vi "Autonomous Independent.vi"() -> ()   [LabVIEW 2015]
doc: "This VI is called when autonomous begins, and will automatically be terminated when autonomous ends. You can carry out timed or sensor driven robot movement independently without needing to return to the caller."
uses:
  <vilib>/Rock Robotics/WPI/Solenoid/WPI_SolenoidValue.ctl
  <vilib>/Rock Robotics/WPI/CAN/TalonSRX/WPI_CANTalonSRX_APIControlMode.ctl
  <vilib>/Rock Robotics/WPI/Utilities/WPI_GetSetVariantRefNum.vi
  <vilib>/Rock Robotics/Network Tables/NT Write Numeric Array.vi
  <vilib>/Rock Robotics/Network Tables/NT Read String.vi
  <vilib>/Rock Robotics/WPI/RobotDrive/WPI_RobotDriveArcadeDrive_Standard(NoSaturation).vi
  <vilib>/Rock Robotics/Network Tables/NT Write Boolean.vi
  <vilib>/Rock Robotics/WPI/Solenoid/WPI_SolenoidSetEnum.vi
  <vilib>/Rock Robotics/Network Tables/NT Read Number.vi
  Distance.vi
panel:
  out "Current Movement, for debugging":T1 {"Y Joystick Value" scale=1.0..-1.0; "X Joystick Value" scale=-1.0..1.0}
  in  "Array of robot movements":T2(array[cluster])=[{"X Joystick Value"=0.39393939393939403, "Y Joystick Value"=0.0, "Delay (sec)"=1.0, "Movement Name"="turn"}, {"X Joystick Value"=-0.3737373737373737, "Y Joystick Value"=0.0, "Delay (sec)"=1.0, "Movement Name"="turn back"}] {"Y Joystick Value" scale=1.0..-1.0; "X Joystick Value" scale=-1.0..1.0}
  # "Be sure to right-click and choose Data Operations>>Make Current Value default if you want to save the array values with the VI"
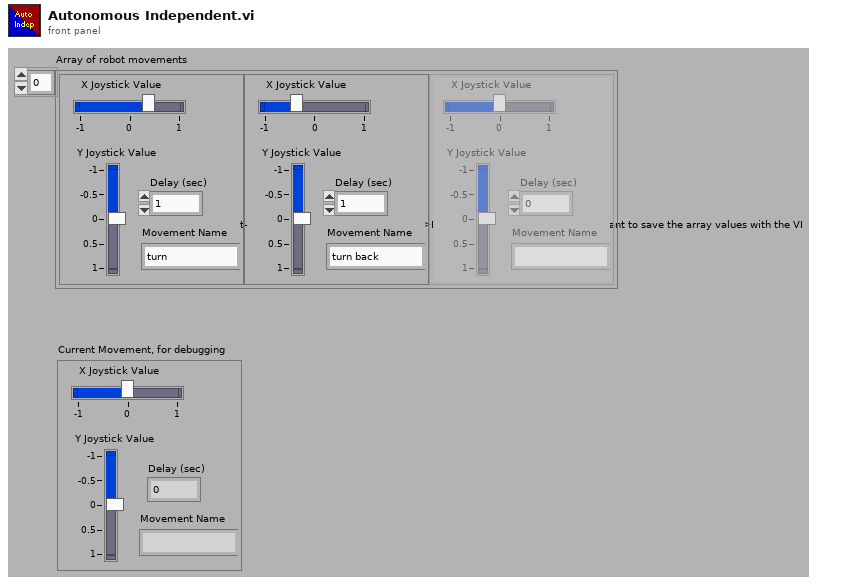
[diagram p1: front panel]
types:
  T1 = cluster{"X Joystick Value":dbl, "Y Joystick Value":dbl, "Delay (sec)":dbl, "Movement Name":string}
  T2 = cluster{"X Joystick Value":dbl, "Y Joystick Value":dbl, "Delay (sec)":dbl, "Movement Name":string}[]
  T3 = typedef "WPI_JoystickDevRef.ctl" = cluster{"Device":T4}
  T4 = typedef "WPI_JoystickDeviceEnum.ctl" = enum16{"USB 0", "USB 1", "USB 2", "USB 3", "USB 4", "USB 5"}
  T5 = typedef "WPI_SolenoidValue.ctl" = enum16{"Off", "On", "Forward", "Reverse"}
  T6 = typedef "WPI_RobotDriveDevRef.ctl" = cluster{"DevStatus":errorcluster, "Motors[]":T7[], "Square Inputs":bool, "Max Output":dbl}
  T7 = typedef "WPI_MotorControlDeviceRef.ctl" = cluster{"DeviceStatus":errorcluster, "Type":T8, "PWM":cluster{"PWM Channel":T9, "DeadBand":T10}, "CAN":cluster{"Device Number":u8, "Control Mode":T11, "Semaphore":T12, "Max Vout":dbl, "TalonSRX Control Mode":T13}, "Invert":bool}
  T8 = typedef "WPI_MotorControlType.ctl" = enum16{"PWM", "CAN", "CANTalonSRX"}
  T9 = typedef "FPGA_DIOPWMChannel.ctl" = enum8{"PWM 0", "PWM 1", "PWM 2", "PWM 3", "PWM 4", "PWM 5", "PWM 6", "PWM 7", "PWM 8", "PWM 9", "PWM MXP 0", "PWM MXP 1", "PWM MXP 2", "PWM MXP 3", "PWM MXP 4", "PWM MXP 5", "PWM MXP 6", "PWM MXP 7", "PWM MXP 8", "PWM MXP 9", "Invalid"}
  T10 = typedef "WPI_PWMDeadband.ctl" = cluster{"Name":string, "maxPositivePwm":i32, "minPositivePwm":i32, "centerPwm":i32, "maxNegativePwm":i32, "minNegativePwm":i32, "angularRange":u16}
  T11 = typedef "WPI_CANJaguar_ControlMode.ctl" = enum8{"Percent VBus", "Current", "Speed", "Position", "Voltage"}
  T12 = typedef "Semaphore RefNum" = refnum<k1>
  T13 = typedef "WPI_CANTalonSRX_APIControlMode.ctl" = enum8{"Percent VBus", "Speed", "Position", "Slave", "Unchanged / Invalid", "Voltage Compensation", "Current", "Motion Profile"}
  T14 = typedef "WPI_SolenoidDevRef.ctl" = cluster{"DevStatus":errorcluster, "Pneumatics Control Module":u8, "Forward Solenoid Channel":T15, "Reverse Solenoid Channel":T15}
  T15 = typedef "WPI_SolenoidChannel.ctl" = enum8{"Solenoid 0", "Solenoid 1", "Solenoid 2", "Solenoid 3", "Solenoid 4", "Solenoid 5", "Solenoid 6", "Solenoid 7", "Invalid"}
  T16 = typedef "WPI_ServoDeviceRef.ctl" = cluster{"DeviceStatus":errorcluster, "PWM Channel":T9, "DeadBand":T10}
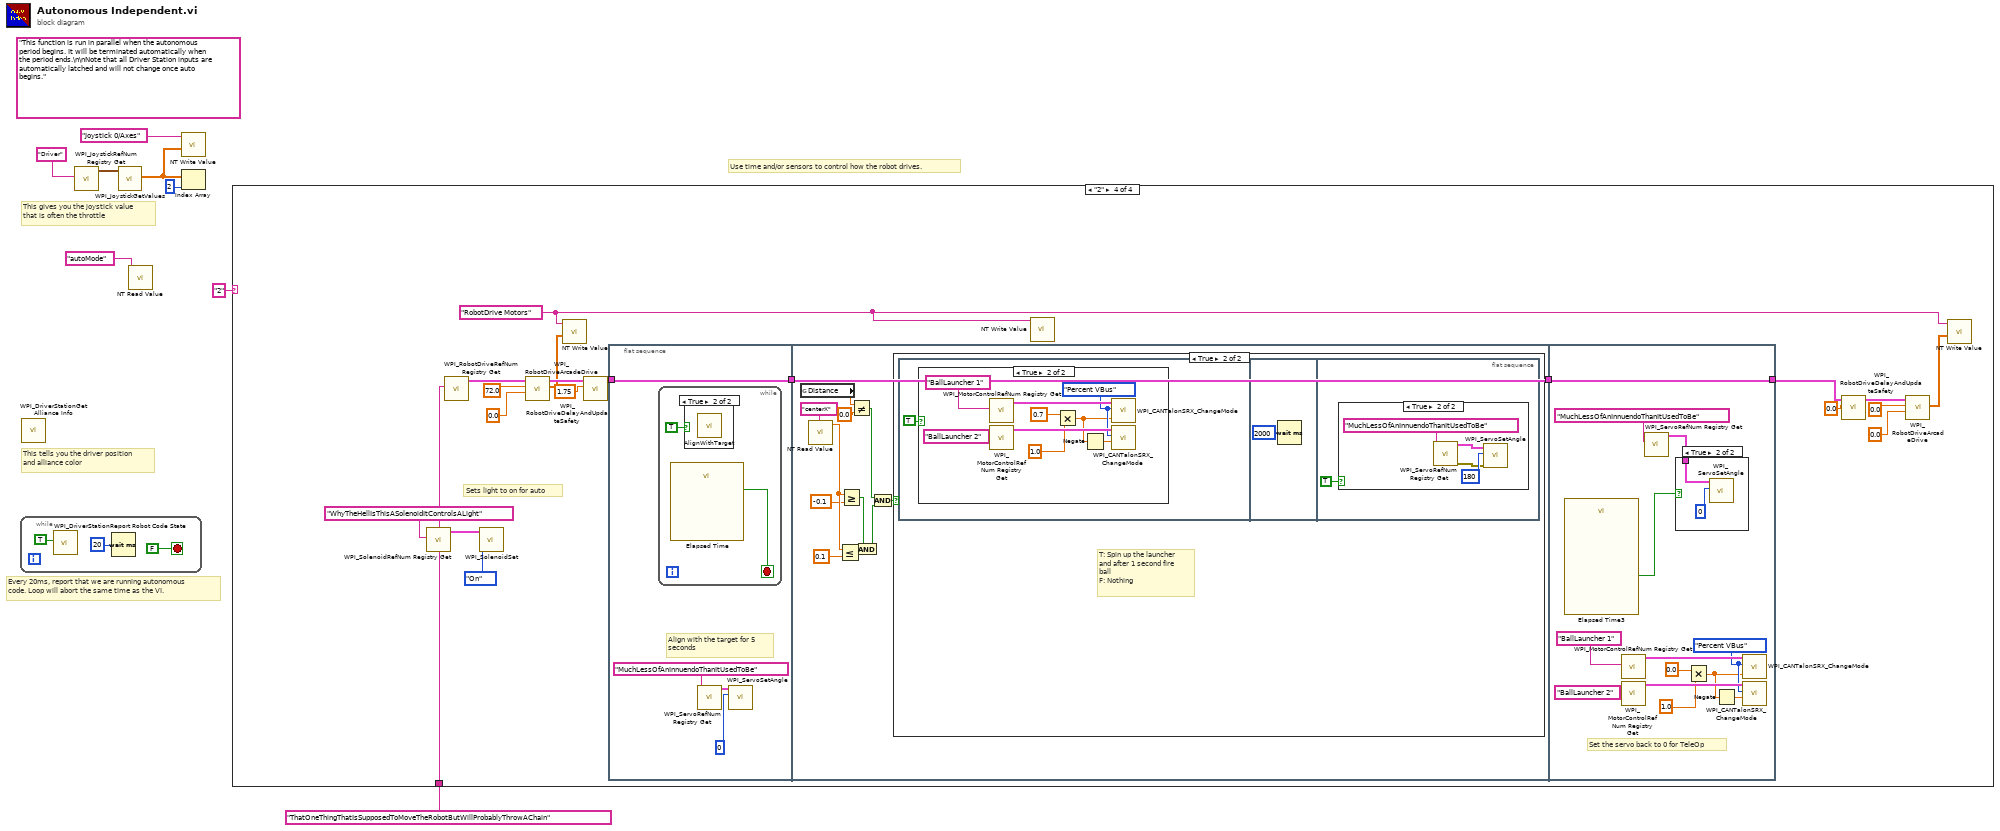
[diagram p0: block diagram]
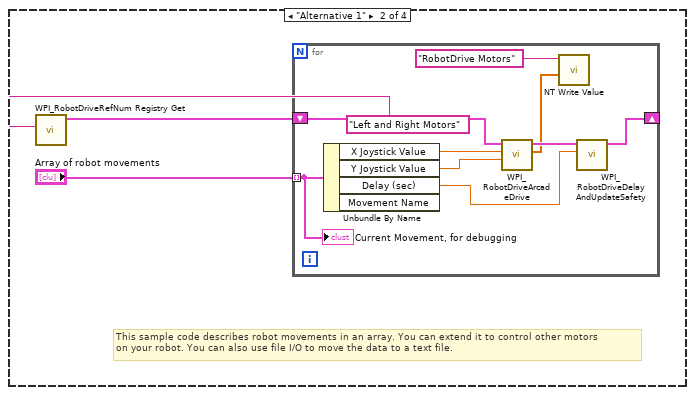
[diagram p3: hidden frame]
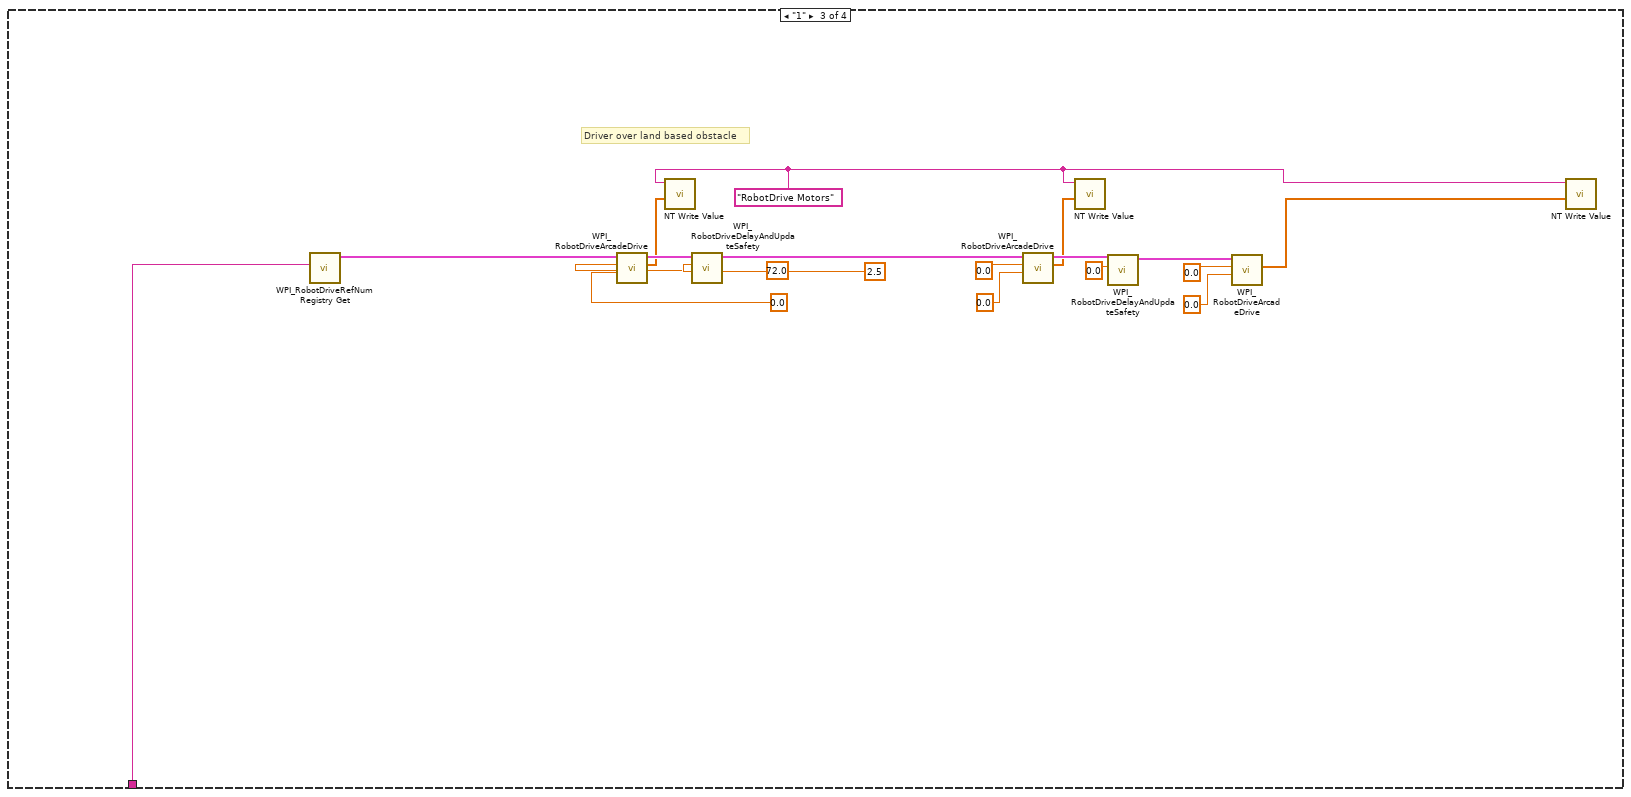
[diagram p4: hidden frame]
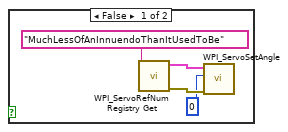
[diagram p8: hidden frame]
diagram:
  (unwired) "This function is run in parallel when the autonomous period begins. It will be terminated automatically when the period ends.\n\nNote that all Driver Station inputs are automatically latched and will not change once auto begins."
  # "Every 20ms, report that we are running autonomous\ncode. Loop will abort the same time as the VI."
  # "This gives you the joystick value\nthat is often the throttle"
  # "Use time and/or sensors to control how the robot drives."
  # "This tells you the driver position\nand alliance color"
  n1 = while {
    stop <- FALSE stop-if-true
    n2 = call <vilib>:"WPI_DriverStationReport Robot Code State.vi"("Autonomous"=TRUE) -> ()  [unwired: 10 in, 1 out]
    n3 = Wait (ms)(milliseconds to wait=u32 20) -> ()  [unwired: 1 out]
  }
  n4 = call <vilib>:"WPI_DriverStationGet Alliance Info.vi"() -> ()  [unwired: 12 out]
  n5 = call <vilib>:"WPI_JoystickRefNum Registry Get.vi"("refnum name"="Driver") -> ("JoystickDevRef"=w7:T3)  [unwired: 1 in, 9 out]
  n6 = call <vilib>:"WPI_JoystickGetValues.vi"("JoystickDevRef"=w7) -> ("Axes"=w5:dbl[])  [unwired: 6 in, 4 out]
  n7 = call-poly <vilib>:"NT Read Value.vi"("Name"="autoMode") -> ()  [unwired: 9 in, 2 out]
  n8 = call-poly <vilib>:"NT Write Value.vi"("Numeric Array"=w5, "Name"="Joystick 0/Axes") -> ()  [unwired: 9 in, 1 out]
  n9 = Index Array(array=w5, index=2) -> ()  [unwired: 1 out]
  n10 = case shown="\"2\"" "2" {
    tunnel: "ThatOneThingThatIsSupposedToMoveTheRobotButWillProbablyThrowAChain" ("refnum name") -> [_ _ w24 w49]
    frame Default {
      # "You can put your main auto here, or you can right-click on the case and make any\nother frame be the default case."
      # "This is the frame that will execute if no selection is made, or if it is not recognized"
    }
    frame "Alternative 1" {
      # "This sample code describes robot movements in an array. You can extend it to control other motors\non your robot. You can also use file I/O to move the data to a text file."
      n11 = call <vilib>:"WPI_RobotDriveRefNum Registry Get.vi"("refnum name"="Left and Right Motors") -> ("RobotDriveDevRef"=w13:T6)  [unwired: 1 in, 9 out]
      n12 = for {
        shift-right: [w21] -> _
        shift-left: w13 -> [w22]
        tunnel: "Array of robot movements" -> [w17] mode=indexing
        n13 = Unbundle By Name(w17) -> ("X Joystick Value"=w20:dbl, "Y Joystick Value"=w19:dbl, "Delay (sec)"=w18:dbl)  [unwired: 1 out]
        n14 = call-poly <vilib>:"WPI_RobotDriveArcadeDrive.vi"("Y axis value"=w19, "X axis value"=w20, "RobotDriveDevRef"=w22) -> ("Motor Values"=w15:dbl[], "RobotDriveDevRef"=w23:T6)  [unwired: 1 in, 6 out]
        n15 = call-poly <vilib>:"NT Write Value.vi"("Numeric Array"=w15, "Name"="RobotDrive Motors") -> ()  [unwired: 9 in, 1 out]
        n16 = call <vilib>:"WPI_RobotDriveDelayAndUpdateSafety.vi"("Delay (s)"=w18, "RobotDriveDevRef"=w23) -> ("RobotDriveDevRef 2"=w21:T6)  [unwired: 8 in, 1 out]
        "Current Movement, for debugging" <- w17
      }
    }
    frame "1" {
      w26 = "RobotDrive Motors" ("Name")
      # "Driver over land based obstacle"
      n17 = call <vilib>:"WPI_RobotDriveRefNum Registry Get.vi"("refnum name"=w24) -> ("RobotDriveDevRef"=w41:T6)  [unwired: 1 in, 9 out]
      n18 = call-poly <vilib>:"WPI_RobotDriveArcadeDrive.vi"("Y axis value"=0.0 ("X axis value"), "X axis value"=72.0, "RobotDriveDevRef"=w41) -> ("Motor Values"=w25:dbl[], "RobotDriveDevRef"=w35:T6)  [unwired: 1 in, 6 out]
      n19 = call-poly <vilib>:"NT Write Value.vi"("Numeric Array"=w25, "Name"=w26) -> ()  [unwired: 9 in, 1 out]
      n20 = call <vilib>:"WPI_RobotDriveDelayAndUpdateSafety.vi"("Delay (s)"=2.5, "RobotDriveDevRef"=w35) -> ("RobotDriveDevRef 2"=w36:T6)  [unwired: 8 in, 1 out]
      n21 = call-poly <vilib>:"WPI_RobotDriveArcadeDrive.vi"("Y axis value"=0.0 ("X axis value"), "X axis value"=0.0, "RobotDriveDevRef"=w36) -> ("Motor Values"=w27:dbl[], "RobotDriveDevRef"=w37:T6)  [unwired: 1 in, 6 out]
      n22 = call-poly <vilib>:"NT Write Value.vi"("Numeric Array"=w27, "Name"=w26) -> ()  [unwired: 9 in, 1 out]
      n23 = call <vilib>:"WPI_RobotDriveDelayAndUpdateSafety.vi"("Delay (s)"=0.0, "RobotDriveDevRef"=w37) -> ("RobotDriveDevRef 2"=w38:T6)  [unwired: 8 in, 1 out]
      n24 = call-poly <vilib>:"WPI_RobotDriveArcadeDrive.vi"("Y axis value"=0.0 ("X axis value"), "X axis value"=0.0, "RobotDriveDevRef"=w38) -> ("Motor Values"=w28:dbl[])  [unwired: 1 in, 7 out]
      n25 = call-poly <vilib>:"NT Write Value.vi"("Numeric Array"=w28, "Name"=w26) -> ()  [unwired: 9 in, 1 out]
    }
    frame "2" {
      w51 = "RobotDrive Motors" ("Name")
      # "Sets light to on for auto"
      n26 = call <vilib>:"WPI_SolenoidRefNum Registry Get.vi"("refnum name"="WhyTheHellIsThisASolenoidItControlsALight") -> ("SolenoidDevRef"=w43:T14)  [unwired: 9 in, 1 out]
      n27 = call <vilib>:"WPI_RobotDriveRefNum Registry Get.vi"("refnum name"=w49) -> ("RobotDriveDevRef"=w61:T6)  [unwired: 1 in, 9 out]
      n28 = call-poly <vilib>:"WPI_SolenoidSet.vi"("Value"=WPI_SolenoidValue."On", "SolenoidDevRef"=w43) -> ()  [unwired: 8 in, 2 out]
      n29 = call-poly <vilib>:"WPI_RobotDriveArcadeDrive.vi"("Y axis value"=0.0 ("X axis value"), "X axis value"=72.0, "RobotDriveDevRef"=w61) -> ("Motor Values"=w50:dbl[], "RobotDriveDevRef"=w57:T6)  [unwired: 1 in, 6 out]
      n30 = call-poly <vilib>:"NT Write Value.vi"("Numeric Array"=w50, "Name"=w51) -> ()  [unwired: 9 in, 1 out]
      n31 = call <vilib>:"WPI_RobotDriveDelayAndUpdateSafety.vi"("Delay (s)"=1.75, "RobotDriveDevRef"=w57) -> ("RobotDriveDevRef 2"=w48:T6)  [unwired: 8 in, 1 out]
      n32 = flat-sequence {
        tunnel: w48 -> [w65]
        tunnel: [w65] -> w46
        tunnel: w46 -> [w79]
        tunnel: [w79] -> w45
        tunnel: [w112] -> w47
        tunnel: w45 -> [w112]
        frame #0 {
          # "Align with the target for 5\nseconds"
          n33 = while {
            stop <- w66 stop-if-true
            n34 = call "Elapsed Time"() -> ("Time has Elapsed"=w66:bool)  [unwired: 12 in, 7 out]
            n35 = case shown="True" TRUE {
              frame False {
              }
              frame True {
                n36 = call "AlignWithTarget.vi"() -> ()  [unwired: 12 in]
              }
            }
          }
          n37 = call <vilib>:"WPI_ServoRefNum Registry Get.vi"("refnum name"="MuchLessOfAnInnuendoThanItUsedToBe") -> ("ServoDeviceRef"=w62:T16)  [unwired: 9 in, 1 out]
          n38 = call <vilib>:"WPI_ServoSetAngle.vi"("Angle"=0, "ServoDeviceRef"=w62) -> ()  [unwired: 8 in, 2 out]
        }
        frame #1 {
          n39 = global read "Distance.vi" "Distance"() -> (w73:dbl)
          n40 = call-poly <vilib>:"NT Read Value.vi"("Name"="centerX") -> ("Numeric"=w77:dbl)  [unwired: 9 in, 1 out]
          n41 = Less Or Equal?(x=w77, y=0.1) -> (x <= y?=w71:bool)
          n42 = Greater Or Equal?(x=w77, y=-0.1) -> (x >= y?=w74:bool)
          n43 = Not Equal?(x=w73, y=0.0) -> (x != y?=w69:bool)
          n44 = And(x=w74, y=w71) -> (x .and. y?=w70:bool)
          n45 = And(x=w69, y=w70) -> (x .and. y?=w68:bool)
          n46 = case shown="True" w68 {
            frame False {
            }
            frame True {
              # "T: Spin up the launcher\nand after 1 second fire\nball\nF: Nothing"
              n47 = flat-sequence {
                frame #0 {
                  n48 = case shown="True" TRUE {
                    frame False {
                    }
                    frame True {
                      w87 = WPI_CANTalonSRX_APIControlMode."Percent VBus" ("Control Mode")
                      n49 = call <vilib>:"WPI_MotorControlRefNum Registry Get.vi"("refnum name"="BallLauncher 1") -> ("MotorControlDevRef"=w88:T7)  [unwired: 9 in, 1 out]
                      n50 = call <vilib>:"WPI_MotorControlRefNum Registry Get.vi"("refnum name"="BallLauncher 2") -> ("MotorControlDevRef"=w89:T7)  [unwired: 9 in, 1 out]
                      n51 = Multiply(x=0.7, y=1.0) -> (x*y=w82:dbl)
                      n52 = Negate(x=w82) -> (-x=w83:dbl)
                      n53 = call <vilib>:"WPI_CANTalonSRX_ChangeMode.vi"("Output"=w82, "Control Mode"=w87, "CAN Talon SRX Ref"=w88) -> ()  [unwired: 7 in, 2 out]
                      n54 = call <vilib>:"WPI_CANTalonSRX_ChangeMode.vi"("Output"=w83, "Control Mode"=w87, "CAN Talon SRX Ref"=w89) -> ()  [unwired: 7 in, 2 out]
                    }
                  }
                }
                frame #1 {
                  n55 = Wait (ms)(milliseconds to wait=u32 2000) -> ()  [unwired: 1 out]
                }
                frame #2 {
                  n56 = case shown="True" TRUE {
                    frame False {
                      n57 = call <vilib>:"WPI_ServoRefNum Registry Get.vi"("refnum name"="MuchLessOfAnInnuendoThanItUsedToBe") -> ("error out"=w93:errorcluster, "ServoDeviceRef"=w94:T16)  [unwired: 9 in]
                      n58 = call <vilib>:"WPI_ServoSetAngle.vi"("error in (no error)"=w93, "Angle"=0, "ServoDeviceRef"=w94) -> ()  [unwired: 7 in, 2 out]
                    }
                    frame True {
                      n59 = call <vilib>:"WPI_ServoRefNum Registry Get.vi"("refnum name"="MuchLessOfAnInnuendoThanItUsedToBe") -> ("error out"=w98:errorcluster, "ServoDeviceRef"=w97:T16)  [unwired: 9 in]
                      n60 = call <vilib>:"WPI_ServoSetAngle.vi"("error in (no error)"=w98, "Angle"=180, "ServoDeviceRef"=w97) -> ()  [unwired: 7 in, 2 out]
                    }
                  }
                }
              }
            }
          }
        }
        frame #2 {
          w106 = WPI_CANTalonSRX_APIControlMode."Percent VBus" ("Control Mode")
          # "Set the servo back to 0 for TeleOp"
          n61 = call "Elapsed Time3"() -> ("Time has Elapsed"=w109:bool)  [unwired: 12 in, 7 out]
          n62 = call <vilib>:"WPI_MotorControlRefNum Registry Get.vi"("refnum name"="BallLauncher 1") -> ("MotorControlDevRef"=w107:T7)  [unwired: 9 in, 1 out]
          n63 = call <vilib>:"WPI_MotorControlRefNum Registry Get.vi"("refnum name"="BallLauncher 2") -> ("MotorControlDevRef"=w108:T7)  [unwired: 9 in, 1 out]
          n64 = call <vilib>:"WPI_ServoRefNum Registry Get.vi"("refnum name"="MuchLessOfAnInnuendoThanItUsedToBe") -> ("ServoDeviceRef"=w110:T16)  [unwired: 9 in, 1 out]
          n65 = case shown="True" w109 {
            tunnel: w110 -> [_ w113]
            frame False {
            }
            frame True {
              n66 = call <vilib>:"WPI_ServoSetAngle.vi"("Angle"=0, "ServoDeviceRef"=w113) -> ()  [unwired: 8 in, 2 out]
            }
          }
          n67 = Multiply(x=0.0, y=1.0) -> (x*y=w101:dbl)
          n68 = Negate(x=w101) -> (-x=w102:dbl)
          n69 = call <vilib>:"WPI_CANTalonSRX_ChangeMode.vi"("Output"=w101, "Control Mode"=w106, "CAN Talon SRX Ref"=w107) -> ()  [unwired: 7 in, 2 out]
          n70 = call <vilib>:"WPI_CANTalonSRX_ChangeMode.vi"("Output"=w102, "Control Mode"=w106, "CAN Talon SRX Ref"=w108) -> ()  [unwired: 7 in, 2 out]
        }
      }
      n71 = call-poly <vilib>:"NT Write Value.vi"("Name"=w51) -> ()  [unwired: 10 in, 1 out]
      n72 = call <vilib>:"WPI_RobotDriveDelayAndUpdateSafety.vi"("Delay (s)"=0.0, "RobotDriveDevRef"=w47) -> ("RobotDriveDevRef 2"=w58:T6)  [unwired: 8 in, 1 out]
      n73 = call-poly <vilib>:"WPI_RobotDriveArcadeDrive.vi"("Y axis value"=0.0 ("X axis value"), "X axis value"=0.0, "RobotDriveDevRef"=w58) -> ("Motor Values"=w52:dbl[])  [unwired: 1 in, 7 out]
      n74 = call-poly <vilib>:"NT Write Value.vi"("Numeric Array"=w52, "Name"=w51) -> ()  [unwired: 9 in, 1 out]
    }
  }
